vi "GetModificationsBitsets.vi"(8 "Error In":errorcluster, 11 "Application Reference":refnum<vi>) -> (0 "Error Out":errorcluster, 3 "DocMods for All Items in Memory":T1(array[cluster]))   [LabVIEW 2013, in "DiscoverCommonTypeDefCallers.lvlib"]
doc: "Searches through all items in memory, belonging to the specified Application Instance, and gets each item's Modification Bitsets, which describe what DocMods have been made since it was last saved."
uses:
  DiscoverCommonTypeDefCallers.lvlib
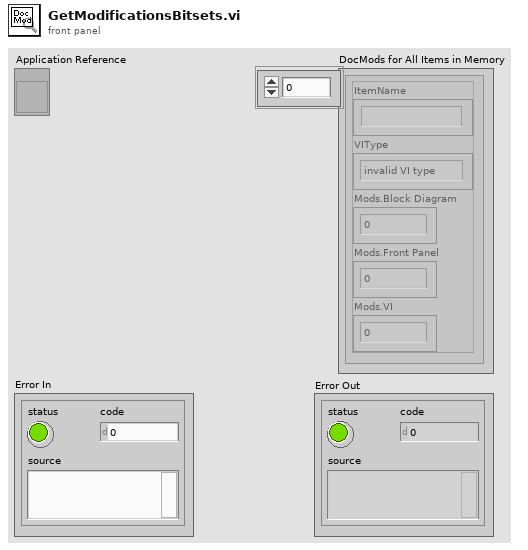
[diagram p1: front panel]
types:
  T1 = cluster{"ItemName":string, "VIType":enum32{"invalid VI type", "Standard VI", "Control VI", "Global VI", "Polymorphic VI", "Configuration VI", "SubSystem", "Facade VI", "Method VI", "Statechart Diagram VI"}, "Mods.Block Diagram":u32, "Mods.Front Panel":u32, "Mods.VI":u64}[]
  T2 = cluster{string, "VIType":enum32{"invalid VI type", "Standard VI", "Control VI", "Global VI", "Polymorphic VI", "Configuration VI", "SubSystem", "Facade VI", "Method VI", "Statechart Diagram VI"}, "Mods.Block Diagram":u32, "Mods.Front Panel":u32, "Mods.VI":u64}[]
  T3 = enum32{"invalid VI type", "Standard VI", "Control VI", "Global VI", "Polymorphic VI", "Configuration VI", "SubSystem", "Facade VI", "Method VI", "Statechart Diagram VI"}
  T4 = cluster{string, "VIType":enum32{"invalid VI type", "Standard VI", "Control VI", "Global VI", "Polymorphic VI", "Configuration VI", "SubSystem", "Facade VI", "Method VI", "Statechart Diagram VI"}, "Mods.Block Diagram":u32, "Mods.Front Panel":u32, "Mods.VI":u64}
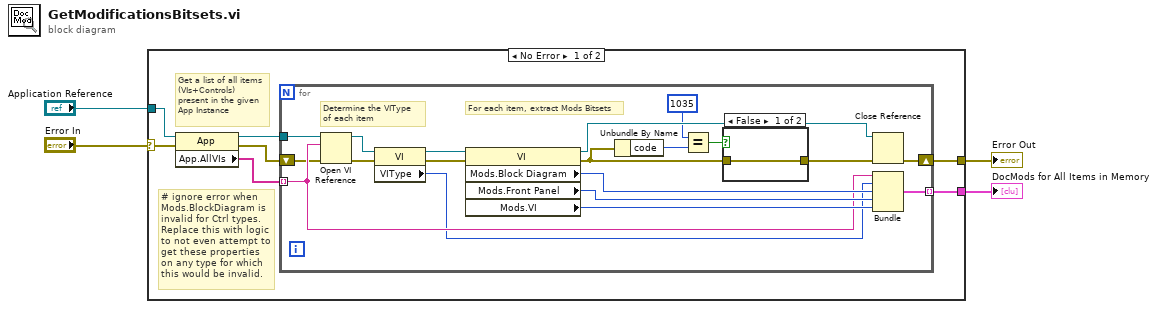
[diagram p0: block diagram]
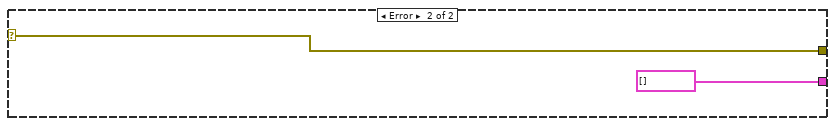
[diagram p3: hidden frame]
diagram:
  n1 = case shown="No Error" "Error In" {
    selector: "Error In" -> [w7 w33]
    tunnel: [w8 w33] -> w2
    tunnel: "Application Reference" -> [w9 _]
    tunnel: [w5 T2 []] -> w1
    frame No Error {
      # "# ignore error when \nMods.BlockDiagram is invalid for Ctrl types.  Replace this with logic to not even attempt to get these properties on any type for which this would be invalid."
      # "Get a list of all items \n(VIs+Controls) present in the given App Instance"
      n2 = property class="App"(reference=w9, error in=w7) -> (reference out=w10:refnum<vi>, error out=w6:errorcluster, "App.AllVIs"=w11:string[])
      n3 = for {
        tunnel: w11 -> [w20] mode=indexing
        tunnel: w10 -> [w29]
        tunnel: [w28] -> w5 mode=indexing
        shift-right: [w27] -> w8
        shift-left: w6 -> [w18]
        # "For each item, extract Mods Bitsets"
        # "Determine the VIType \nof each item"
        n4 = Open VI Reference(application reference (local)=w29, vi path=w20, error in (no error)=w18) -> (vi reference=w26:refnum<vi>, error out=w30:errorcluster)  [unwired: 3 in]
        n5 = property class="VI"(reference=w26, error in=w30) -> (reference out=w24:refnum<vi>, error out=w25:errorcluster, "VIType"=w19:T3)
        n6 = property class="VI"(reference=w24, error in=w25) -> (reference out=w17:refnum<vi>, error out=w14:errorcluster, "Mods.Block Diagram"=w23:u32, "Mods.Front Panel"=w21:u32, "Mods.VI"=w22:u64)
        n7 = Unbundle By Name(w14) -> ("code"=w16:i32)
        n8 = Equal?(x=1035 ("Code to filter"), y=w16) -> (x = y?=w15:bool)
        n9 = case shown="False" w15 {
          tunnel: [w31 _] -> w12
          tunnel: w14 -> [w31 _]
          frame False {
          }
          frame True {
          }
        }
        n10 = Close Reference(reference=w17, error in (no error)=w12) -> (error out=w27:errorcluster)
        n11 = Bundle(w20, "VIType"=w19, "Mods.Block Diagram"=w23, "Mods.Front Panel"=w21, "Mods.VI"=w22) -> (w28:T4)  [unwired: 1 in]
      }
    }
    frame Error {
    }
  }
  "Error Out" <- w2
  "DocMods for All Items in Memory" <- w1
